vi "Halvorsen_ECD4_Fast.vi"(0 "tolerance":dbl=1e-13, 1 "Error Analysis":u16(ring)=4 items=["Max", "Max_Norm", "Norm", "Last Value", "Last Constant"], 3 "Шаг h, с":dbl=0.01, 4 "k":i32=4, 5 "Время, с":dbl=30.0, 7 "Hmax":dbl=1.0, 8 "b":dbl[](array[numeric])=[1.4, 1.4, 1.4], 10 "last_point_Thomas":dbl[](array[numeric])=[2.3727475682665875, 0.23609824454436878, 0.4447912442126299], 13 "Hmin":dbl=0.001, 15 "Points count":i32=2, 18 "n":i32[](array[numeric])=[2, 4, 6, 8, 10, 12, 14, 16, 18, 20, 22], 19 "Ext.Type":u16(ring) items=["FNode", "MathScript", "ECD8 Arrays", "ECD8 Fnode", "ECD8 FnodeDiv", "FNode Exp"]) -> (6 "Elapsed Time":dbl=0.006700851644382055, 12 "Number of steps":i32=211, 14 "Error Estimation":dbl=1.5745409996203077e-13, 17 "Rejected steps":i32=3)   [LabVIEW 2016]
uses:
  <vilib>/Analysis/_algsub.llb/Real Vector Norm.vi
  <vilib>/Analysis/5stat.llb/RMS (DBL).vi
  <vilib>/Analysis/NI_AALBase.lvlib
  <vilib>/Analysis/NI_AALPro.lvlib
panel:
  in  "Initial Conditions":dbl[](array[numeric])=[1.0, 0.0, 1.0]
  out "Last Value Reference":dbl[](array[numeric])=[2.3727475682668593, 0.2360982445442987, 0.44479124421215666] format="%#_15f"
  out "Rejected Steps":i32[](graph)=[0, 0, 0, 0, 0, 0, 0, 0, 0, 0, 0, 0, 0, 0, 0, 0, 0, 0, 0, 0, 0, 0, 0, 0, 0, 0, 0, 0, 0, 0, 0, 0, 0, 0, 0, 0, 0, 0, 0, 0, 0, 0, 0, 0, 0, 0, 0, 0, 0, 0, 0, 1, 0, 0, 0, 0, 0, 0, 0, 0, 0, 0, 0, 0, 0, 0, 0, 0, 0, 0, 0, 0, 0, 0, 0, 0, 0, 0, 0, 0, 0, 0, 0, 0, 0, 0, 1, 0, 0, 0, 0, 0, 0, 0, 0, 0, 0, 0, 0, 0, 0, 0, 0, 0, 0, 0, 0, 0, 0, 0, 0, 0, 0, 0, 0, 0, 0, 0, 0, 0, 0, 0, 0, 0, 0, 0, 0, 0, 0, 0, 0, 0, 0, 0, 0, 0, 0, 0, 0, 0, 0, 0, 0, 0, 0, 0, 0, 0, 0, 0, 0, 0, 0, 0, 0, 0, 0, 0, 0, 0, 0, 0, 0, 0, 0, 0, 0, 0, 0, 0, 0, 0, 0, 0, 0, 0, 0, 0, 0, 0, 0, 0, 0, 0, 0, 0, 0, 0, 1, 0, 0, 0, 0, 0, 0, 0, 0, 0, 0, 0, 0, 0, 0, 0, 0, 0, 0, 0, 0, 0, 0, 0]
  out "Last Value":dbl[](array[numeric])=[2.3727475682664667, 0.23609824454430522, 0.4447912442127084] format="%#_15f"
  out "Step time variation":dbl[](graph)=[0.006685207197733689, 0.006716496091030422]
  out "Real Error":dbl[][](graph)=[[0.0, 0.0, 0.0], [9.992007221626409e-16, 1.3877787807814457e-17, 4.6629367034256575e-15], [2.4424906541753444e-15, 3.122502256758253e-17, 6.661338147750939e-15], [-1.2212453270876722e-15, 2.914335439641036e-16, 5.551115123125783e-15], [-5.551115123125783e-15, -5.551115123125783e-17, 2.886579864025407e-15], [-5.10702591327572e-15, 2.7755575615628914e-16, 7.327471962526033e-15], [-7.771561172376096e-15, 1.1657341758564144e-15, 8.881784197001252e-15], [-6.661338147750939e-15, 2.886579864025407e-15, 9.103828801926284e-15], [-9.547918011776346e-15, -2.220446049250313e-16, 9.325873406851315e-15], [-8.215650382226158e-15, 2.886579864025407e-15, 1.1324274851176597e-14], [-7.771561172376096e-15, 2.6645352591003757e-15, 1.5987211554602254e-14], [-1.176836406102666e-14, 1.7763568394002505e-15, 7.327471962526033e-15], [-1.2878587085651816e-14, -1.5543122344752192e-15, 2.886579864025407e-15], [-1.1546319456101628e-14, 1.9984014443252818e-15, 9.769962616701378e-15], [-1.354472090042691e-14, -8.881784197001252e-16, 6.217248937900877e-15], [-2.1316282072803006e-14, -6.661338147750939e-15, 0.0], [-1.4654943925052066e-14, -4.218847493575595e-15, 8.881784197001252e-16], [-1.9539925233402755e-14, -6.661338147750939e-15, 4.884981308350689e-15], [-1.7763568394002505e-14, -1.1102230246251565e-14, 1.2434497875801753e-14], [-1.4654943925052066e-14, -1.3100631690576847e-14, 1.3766765505351941e-14], [-2.886579864025407e-14, -2.220446049250313e-14, 1.4210854715202004e-14], [-2.708944180085382e-14, -2.9976021664879227e-14, 2.1316282072803006e-14], [-3.1530333899354446e-14, -3.042011087472929e-14, 1.6431300764452317e-14], [-3.1530333899354446e-14, -3.219646771412954e-14, 1.8207657603852567e-14], [-3.5083047578154947e-14, -4.1522341120980855e-14, 2.353672812205332e-14], [-3.597122599785507e-14, -4.107825191113079e-14, 2.531308496145357e-14], [-3.6415315207705135e-14, -4.285460875053104e-14, 3.1530333899354446e-14], [-3.1530333899354446e-14, -4.529709940470639e-14, 3.241851231905457e-14], [-1.9539925233402755e-14, -4.285460875053104e-14, 2.708944180085382e-14], [-1.509903313490213e-14, -4.39648317751562e-14, 3.108624468950438e-14], [-2.398081733190338e-14, -4.973799150320701e-14, 2.708944180085382e-14], [-2.398081733190338e-14, -5.5067062021407764e-14, 3.597122599785507e-14], [-1.509903313490213e-14, -5.81756864903582e-14, 3.907985046680551e-14], [-2.7977620220553945e-14, -6.439293542825908e-14, 3.3306690738754696e-14], [-8.881784197001252e-15, -5.595524044110789e-14, 4.218847493575595e-14], [-9.769962616701378e-15, -5.3290705182007514e-14, 3.9968028886505635e-14], [-1.9539925233402755e-14, -5.950795411990839e-14, 3.574918139293004e-14], [-1.0658141036401503e-14, -6.261657858885883e-14, 3.68594044175552e-14], [-5.773159728050814e-15, -7.149836278586008e-14, 3.108624468950438e-14], [8.43769498715119e-15, -7.149836278586008e-14, 3.26405569239796e-14], [9.769962616701378e-15, -6.794564910705958e-14, 2.4202861936828413e-14], [1.7319479184152442e-14, -6.17284001691587e-14, 2.6645352591003757e-14], [2.1760371282653068e-14, -6.217248937900877e-14, 2.2648549702353193e-14], [2.531308496145357e-14, -5.551115123125783e-14, 2.731148640577885e-14], [2.6201263381153694e-14, -7.016609515630989e-14, 1.7985612998927536e-14], [4.218847493575595e-14, -7.283063041541027e-14, 1.2323475573339238e-14], [5.3734794391857577e-14, -7.327471962526033e-14, 6.328271240363392e-15], [6.394884621840902e-14, -6.972200594645983e-14, -2.1094237467877974e-15], [7.016609515630989e-14, -7.593925488436071e-14, -1.3766765505351941e-14], [8.304468224196171e-14, -6.616929226765933e-14, -2.2426505097428162e-14], [1.021405182655144e-13, -6.661338147750939e-14, -3.552713678800501e-14], [1.0791367799356522e-13, -6.616929226765933e-14, -5.1736392947532295e-14], [1.1501910535116622e-13, -5.1958437552457326e-14, -6.361577931102147e-14], [1.2256862191861728e-13, -3.952393967665557e-14, -7.51620987671231e-14], [1.318944953254686e-13, -3.907985046680551e-14, -8.304468224196171e-14], [1.3233858453531866e-13, -5.684341886080802e-14, -9.192646643896296e-14], [1.2789769243681803e-13, -7.904787935331115e-14, -9.880984919163893e-14], [1.361133428190442e-13, -7.815970093361102e-14, -1.0724754417879012e-13], [1.3566925360919413e-13, -8.08242361927114e-14, -1.1546319456101628e-13], [1.3811174426336947e-13, -8.260059303211165e-14, -1.1834977442504169e-13], [1.4477308241112041e-13, -7.638334409421077e-14, -1.0702549957386509e-13], [1.4588330543574557e-13, -6.661338147750939e-14, -1.0391687510491465e-13], [1.4432899320127035e-13, -4.796163466380676e-14, -9.947598300641403e-14], [1.3566925360919413e-13, -6.039613253960852e-14, -9.237055564881302e-14], [1.34781075189494e-13, -6.306066779870889e-14, -7.771561172376096e-14], [1.3433698597964394e-13, -4.1744385725905886e-14, -6.572520305780927e-14], [1.2756462552943049e-13, -5.3290705182007514e-14, -6.039613253960852e-14], [1.283417816466681e-13, -4.529709940470639e-14, -5.10702591327572e-14], [1.2784218128558678e-13, -4.1744385725905886e-14, -2.7533531010703882e-14], [1.2423395645555502e-13, -4.3520742565306136e-14, -1.865174681370263e-14], [1.2059797604990763e-13, -5.240252676230739e-14, -1.2434497875801753e-14], [1.168370955539899e-13, -5.240252676230739e-14, 7.549516567451064e-15], [1.1368683772161603e-13, -4.973799150320701e-14, 2.6645352591003757e-14], [1.1013412404281553e-13, -2.930988785010413e-14, 4.618527782440651e-14], [1.0680345496894006e-13, -6.217248937900877e-14, 5.573319583618286e-14], [1.0169642905566434e-13, -7.37188088351104e-14, 7.038813976123492e-14], [9.348077867343818e-14, -6.661338147750939e-14, 8.126832540256146e-14], [8.926193117986259e-14, -7.105427357601002e-14, 8.72635297355373e-14], [8.004708007547379e-14, -5.1514348342607263e-14, 9.814371537686384e-14], [7.527312106958561e-14, -6.661338147750939e-14, 9.792167077193881e-14], [6.750155989720952e-14, -3.197442310920451e-14, 1.0458300891968975e-13], [6.283862319378386e-14, -4.796163466380676e-14, 1.028066520802895e-13], [5.417888360170764e-14, -2.4868995751603507e-14, 1.0624834345662748e-13], [4.9960036108132044e-14, -1.7763568394002505e-15, 1.0802470029602773e-13], [5.484501741648273e-14, 8.881784197001252e-15, 1.0758061108617767e-13], [5.5067062021407764e-14, 2.842170943040401e-14, 1.0608181000293371e-13], [6.217248937900877e-14, 1.5987211554602254e-14, 1.0330625244137082e-13], [6.750155989720952e-14, 3.8191672047105385e-14, 1.010788674982166e-13], [7.194245199571014e-14, 3.9968028886505635e-14, 9.781064846947629e-14], [6.52811138479592e-14, 6.838973831690964e-14, 9.320322291728189e-14], [6.039613253960852e-14, 9.769962616701378e-14, 8.709699628184353e-14], [7.016609515630989e-14, 1.199040866595169e-13, 8.115730310009894e-14], [7.815970093361102e-14, 1.1191048088221578e-13, 7.494005416219807e-14], [8.482103908136196e-14, 1.0302869668521453e-13, 6.661338147750939e-14], [9.414691248821327e-14, 8.43769498715119e-14, 6.139533326177116e-14], [1.0347278589506459e-13, 7.904787935331115e-14, 5.4289905904170155e-14], [9.947598300641403e-14, 7.283063041541027e-14, 4.5630166312093934e-14], [8.482103908136196e-14, 9.769962616701378e-14, 3.26405569239796e-14], [8.748557434046234e-14, 1.0302869668521453e-13, 2.4202861936828413e-14], [7.505107646466058e-14, 9.325873406851315e-14, 1.4876988529977098e-14], [7.815970093361102e-14, 8.393286066166183e-14, 4.6629367034256575e-15], [7.327471962526033e-14, 8.304468224196171e-14, -2.886579864025407e-15], [6.616929226765933e-14, 7.815970093361102e-14, -8.215650382226158e-15], [6.394884621840902e-14, 6.394884621840902e-14, -1.3100631690576847e-14], [5.773159728050814e-14, 5.595524044110789e-14, -2.1538326677728037e-14], [3.907985046680551e-14, 5.3290705182007514e-14, -2.2426505097428162e-14], [3.552713678800501e-14, 4.529709940470639e-14, -2.19824158875781e-14], [3.419486915845482e-14, 2.6645352591003757e-14, -2.0650148258027912e-14], [3.863576125695545e-14, 2.531308496145357e-14, -2.375877272697835e-14], [2.1760371282653068e-14, 3.4638958368304884e-14, -3.2862601528904634e-14], [1.687538997430238e-14, 2.353672812205332e-14, -2.2870594307278225e-14], [3.9968028886505635e-15, 3.064215547965432e-14, -2.708944180085382e-14], [6.661338147750939e-16, 3.1308289294429414e-14, -2.5091040356528538e-14], [1.3322676295501878e-15, 2.708944180085382e-14, -1.7541523789077473e-14], [-3.9968028886505635e-15, 2.7977620220553945e-14, -2.2426505097428162e-14], [-4.440892098500626e-16, 2.7755575615628914e-14, -2.020605904817785e-14], [-2.6645352591003757e-15, 3.086420008457935e-14, -3.1530333899354446e-14], [3.552713678800501e-15, 2.6201263381153694e-14, -2.4424906541753444e-14], [5.329070518200751e-15, 2.7755575615628914e-14, -1.9984014443252818e-14], [8.659739592076221e-15, 2.6756374893466273e-14, -1.687538997430238e-14], [8.43769498715119e-15, 3.175237850427948e-14, -3.2862601528904634e-14], [9.547918011776346e-15, 3.4638958368304884e-14, -3.108624468950438e-14], [1.7985612998927536e-14, 3.26405569239796e-14, -2.7533531010703882e-14], [2.1871393585115584e-14, 3.2862601528904634e-14, -1.865174681370263e-14], [2.7478019859472624e-14, 3.275157922644212e-14, -9.325873406851315e-15], [3.325117958752344e-14, 3.0309088572266774e-14, 4.440892098500626e-15], [3.6137759451548845e-14, 2.7533531010703882e-14, 1.1102230246251565e-14], [3.902433931557425e-14, 2.525757381022231e-14, 1.6431300764452317e-14], [4.1799896877137144e-14, 2.2065682614424986e-14, 2.1760371282653068e-14], [4.3770542745846797e-14, 1.940114735532461e-14, 1.7319479184152442e-14], [4.601874437071274e-14, 1.6014967130217883e-14, 2.6201263381153694e-14], [4.718447854656915e-14, 1.2692971673722298e-14, 2.4424906541753444e-14], [4.835021272242557e-14, 7.827072323607354e-15, 3.774758283725532e-14], [4.85722573273506e-14, 9.43689570931383e-16, 4.6629367034256575e-14], [4.7600812180803587e-14, -5.773159728050814e-15, 5.3290705182007514e-14], [4.696243394164412e-14, -1.3877787807814457e-14, 7.327471962526033e-14], [4.4353409833775004e-14, -2.4369395390522186e-14, 8.215650382226158e-14], [3.835820550079916e-14, -3.652633751016765e-14, 8.659739592076221e-14], [3.36952687973735e-14, -4.7406523151494184e-14, 8.570921750106208e-14], [2.531308496145357e-14, -5.81756864903582e-14, 8.615330671091215e-14], [1.8540724511240114e-14, -6.872280522429719e-14, 9.192646643896296e-14], [1.1324274851176597e-14, -7.815970093361102e-14, 9.50350909079134e-14], [4.773959005888173e-15, -9.092726571680032e-14, 1.0391687510491465e-13], [-2.1094237467877974e-15, -1.0402789740737717e-13, 1.1723955140041653e-13], [-1.5765166949677223e-14, -1.2312373343092986e-13, 1.1857181902996672e-13], [-3.2862601528904634e-14, -1.4199752484955752e-13, 1.2079226507921703e-13], [-4.463096558993129e-14, -1.5831780331154732e-13, 1.2789769243681803e-13], [-6.283862319378386e-14, -1.7563728249569976e-13, 1.3322676295501878e-13], [-8.038014698286133e-14, -1.9340085088970227e-13, 1.2434497875801753e-13], [-1.0591527654923993e-13, -2.0794477251229182e-13, 1.0702549957386509e-13], [-1.383337888682945e-13, -2.199351811782435e-13, 8.570921750106208e-14], [-1.6653345369377348e-13, -2.2687407508215074e-13, 8.704148513061227e-14], [-1.949551631241775e-13, -2.3397950243975174e-13, 8.970602038971265e-14], [-2.2648549702353193e-13, -2.410571742217371e-13, 9.992007221626409e-14], [-2.6334490144108713e-13, -2.4702462297909733e-13, 8.171241461241152e-14], [-2.9265478929119126e-13, -2.50716114535976e-13, 8.970602038971265e-14], [-3.277378368693462e-13, -2.545741395465484e-13, 1.0036416142611415e-13], [-3.597122599785507e-13, -2.581268532253489e-13, 1.163513729807164e-13], [-3.8413716652030416e-13, -2.602362769721367e-13, 1.1546319456101628e-13], [-4.078959392472825e-13, -2.62234678416462e-13, 1.199040866595169e-13], [-4.289901767151605e-13, -2.62234678416462e-13, 9.059419880941277e-14], [-4.511946372076636e-13, -2.575717417130363e-13, 5.5067062021407764e-14], [-4.662936703425657e-13, -2.552402733613235e-13, 7.105427357601002e-15], [-4.745093207247919e-13, -2.5268676040468563e-13, -4.085620730620576e-14], [-4.815037257799304e-13, -2.489120021209601e-13, -8.08242361927114e-14], [-4.833911049217932e-13, -2.502442697505103e-13, -1.1457501614131615e-13], [-4.843903056439558e-13, -2.475797344914099e-13, -1.4832579608992091e-13], [-4.796163466380676e-13, -2.5224267119483557e-13, -1.865174681370263e-13], [-4.726219415829291e-13, -2.4846791291111003e-13, -2.5845992013273644e-13], [-4.62907490117459e-13, -2.475797344914099e-13, -3.090860900556436e-13], [-4.5086157030027607e-13, -2.4003021792395884e-13, -3.9523939676655573e-13], [-4.3623438195083963e-13, -2.313704783318826e-13, -4.4231285301066237e-13], [-4.1983083676200295e-13, -2.2515322939398175e-13, -4.627409566637652e-13], [-3.990696662015125e-13, -2.0028423364237824e-13, -5.160316618457728e-13], [-3.79585252119341e-13, -1.6786572132332367e-13, -5.586642259913788e-13], [-3.6270986214503864e-13, -1.341149413747189e-13, -6.048495038157853e-13], [-3.446132268436486e-13, -8.570921750106208e-14, -6.421529974431905e-13], [-3.326228181776969e-13, -1.865174681370263e-14, -6.679101716144942e-13], [-3.3284486278262193e-13, 6.616929226765933e-14, -6.918909889463976e-13], [-3.398392678377604e-13, 1.7053025658242404e-13, -7.291944825738028e-13], [-3.6348701826227625e-13, 2.8466118351389014e-13, -7.633893517322576e-13], [-4.050093593832571e-13, 4.0234482412415673e-13, -7.709388682997087e-13], [-4.531930386519889e-13, 5.258016244624741e-13, -7.931433287922118e-13], [-5.131450819817474e-13, 6.346034808757395e-13, -8.109068971862143e-13], [-5.799805080641818e-13, 7.371880883511039e-13, -8.326672684688674e-13], [-6.459277557269161e-13, 8.175682353339653e-13, -8.402167850363185e-13], [-7.001066393286237e-13, 8.921752225887758e-13, -8.624212455288216e-13], [-7.502887200416808e-13, 9.374723219934822e-13, -8.557599073810707e-13], [-7.913669719528116e-13, 9.832135106080386e-13, -8.419931418757187e-13], [-8.022471575941381e-13, 1.007194327939942e-12, -8.231193504570911e-13], [-8.033573806187633e-13, 1.0158540675320182e-12, -7.902567489281864e-13], [-7.902567489281864e-13, 1.0114131754335176e-12, -7.538414337204813e-13], [-7.620570841027074e-13, 9.9253938401489e-13, -7.049916206369744e-13], [-7.225331444260519e-13, 9.65227897609111e-13, -6.481482017761664e-13], [-6.497025140106416e-13, 9.319212068703564e-13, -5.915268275202834e-13], [-5.644373857194296e-13, 8.967271369897389e-13, -5.426770144367765e-13], [-4.902744876744691e-13, 8.524292383071952e-13, -4.947153797729698e-13], [-4.1966430330830917e-13, 8.066880496926387e-13, -4.455324997820753e-13], [-3.299582829185965e-13, 7.603917495657697e-13, -4.034550471487819e-13], [-2.4158453015843406e-13, 7.093770015842438e-13, -3.672617765460018e-13], [-1.580957587066223e-13, 6.575850974854802e-13, -3.377298440909726e-13], [-5.062616992290714e-14, 6.074585279236544e-13, -3.207434318142077e-13], [4.263256414560601e-14, 5.561107130347409e-13, -3.161360062620133e-13], [1.283417816466681e-13, 5.040690087554367e-13, -3.2229774404868294e-13], [2.0472512574087887e-13, 4.4883541328033516e-13, -3.3889557826682903e-13], [2.6556534749033744e-13, 3.8989644846054716e-13, -3.6187719487656977e-13], [3.157474282033945e-13, 3.2633618030075695e-13, -3.9163117193652397e-13], [3.4638958368304884e-13, 2.5711377471537844e-13, -4.2539582967293654e-13], [3.859135233597044e-13, 1.8274270985330077e-13, -4.619638005465276e-13], [3.956834859764058e-13, 1.0211276268989877e-13, -5.017652959793395e-13], [3.943512183468556e-13, 1.712519015484304e-14, -5.417333248658451e-13], [3.9257486150745535e-13, -6.522560269672795e-15, -5.517253320874715e-13]]
  out "Step Variation":dbl[](graph)=[0.01, 0.023360677996708375, 0.05456832298719971, 0.10609865677759227, 0.14228685817737252, 0.1433521858258461, 0.13912016368248273, 0.1353848978239948, 0.1348787008039935, 0.13789794946241468, 0.14183965168589427, 0.1389018246685753, 0.13480655511664044, 0.1352937955188443, 0.14083631069515853, 0.15054302015732818, 0.15354936807919295, 0.15012909437801925, 0.15233158646615488, 0.16195221907261806, 0.1859888941921947, 0.19081476436473468, 0.16882309271455131, 0.16110756221534117, 0.15751551557922944, 0.15515566263423652, 0.1537986192378969, 0.15441647648808968, 0.15703348889728966, 0.16223661244468615, 0.16523261129770903, 0.1575552847464681, 0.14923788348804234, 0.14420094794209656, 0.14333043693757236, 0.14305599030596625, 0.1451932462186197, 0.1484158449420317, 0.15105915525521163, 0.15267209809470114, 0.15128993514268424, 0.1473508980423149, 0.14417110851040923, 0.14259673520710134, 0.1438612133690481, 0.14531637887383417, 0.1489824606828707, 0.15335475631763087, 0.1583176965097996, 0.1645478155214016, 0.1758092639086622, 0.1662066741033067, 0.1471159764326851, 0.1367282453140493, 0.13035995246764745, 0.12717631788307218, 0.12761153374775996, 0.13218596626534898, 0.1395535058928262, 0.1359873295729682, 0.1279072153561344, 0.12677916749215723, 0.13020671862805994, 0.14054161466738815, 0.14955735646322033, 0.1422870923630447, 0.13947030152822443, 0.1425137619209431, 0.14861606101153554, 0.15532871545503943, 0.16063336757924904, 0.16156986300229476, 0.15420612102053258, 0.1452179402961989, 0.13922466410526793, 0.13618167321476882, 0.13478266135199252, 0.13483812596599676, 0.1368349300001295, 0.1419973850154061, 0.1492979861408155, 0.1630793688516221, 0.1698407314481118, 0.1660731905847401, 0.16476318145002147, 0.17023890658894714, 0.17794557645431167, 0.15417389965318076, 0.14164279375448932, 0.13699467420144448, 0.14016009907464672, 0.14454490990645175, 0.13059324979206005, 0.12253189529550425, 0.1201054691030008, 0.12208443771041655, 0.1268938879187612, 0.13135378363117228, 0.13149948182226284, 0.13091376094679263, 0.1330358218423598, 0.13498918498691118, 0.134693349945233, 0.1332797222087208, 0.1327545271092479, 0.132096286825721, 0.12572137094659197, 0.11851952468371733, 0.11440885990029541, 0.11408975301000251, 0.11845938663500437, 0.1251657972697687, 0.11744274061194553, 0.11116682029079179, 0.11109183499278635, 0.11563403836804881, 0.12843660419635064, 0.1340781134326106, 0.12308149559662285, 0.121269099319311, 0.12397097627136096, 0.1310044455798987, 0.14256647877408143, 0.15612558917515526, 0.1559767909870482, 0.1516395775231047, 0.15061109839379794, 0.15131873674559188, 0.15303037557568117, 0.15537721190750214, 0.15765681556191427, 0.16079007115021313, 0.16385724409617003, 0.167421072233169, 0.1705799765382728, 0.17136763902468344, 0.16834897464401802, 0.16344776456145238, 0.15906244550119522, 0.15566817976109593, 0.15384896253401684, 0.15397043019905826, 0.15647351646131896, 0.162778286355558, 0.17312680493100446, 0.17301716184922508, 0.16211595058856945, 0.156911165553237, 0.1572960348891089, 0.1621783969662183, 0.16988978762207912, 0.1676270098812039, 0.15942001429121724, 0.15559916575909497, 0.15555986759313123, 0.1559835273600667, 0.1507770825869849, 0.14519292747781615, 0.1433104622596264, 0.14815336806507956, 0.1568099336449324, 0.14420289290775362, 0.1355769624824643, 0.1343908665158623, 0.1370423708466838, 0.13629799178478536, 0.12965040110128848, 0.12412220297706678, 0.12165762374815889, 0.12108927036893419, 0.12229191822314137, 0.1249944269950167, 0.12751852881829193, 0.12884740536200978, 0.13001514453120236, 0.13295980367479468, 0.13840032844181696, 0.14741206326398376, 0.1600655659399263, 0.16646454630924873, 0.15939804241832492, 0.1539502667088633, 0.15155926283142948, 0.14757446042942224, 0.13541405056970915, 0.1283102292451462, 0.12813003375040924, 0.14225861622847752, 0.1379919455900096, 0.11953673896290772, 0.1151409444583287, 0.11697515743692918, 0.12465131478568296, 0.13338397902464036, 0.1250281665230314, 0.12183451816436883, 0.12393101719177703, 0.12916307570698296, 0.13739294100052019, 0.14654556714718814, 0.15040081725418902, 0.15046036573986937, 0.15011424337824786, 0.15087157526841347, 0.1526751737514233, 0.1550753687685979, 0.15872031300368974, 0.16265538427893264, 0.16696159138984856, 0.17040820371236481, 0.04907266583554204, 0.0]
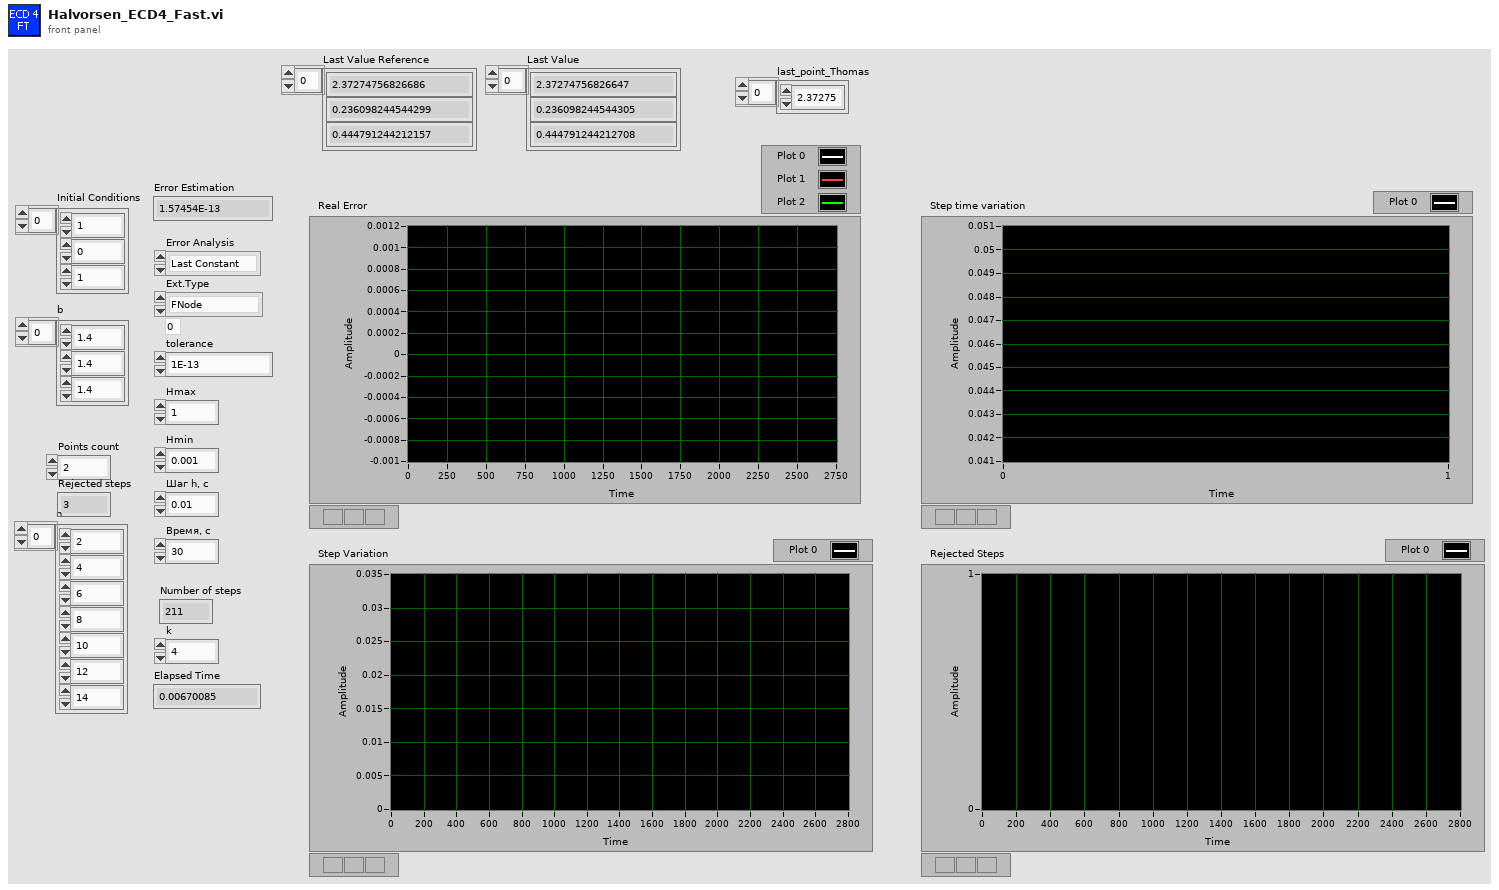
[diagram p1: front panel]
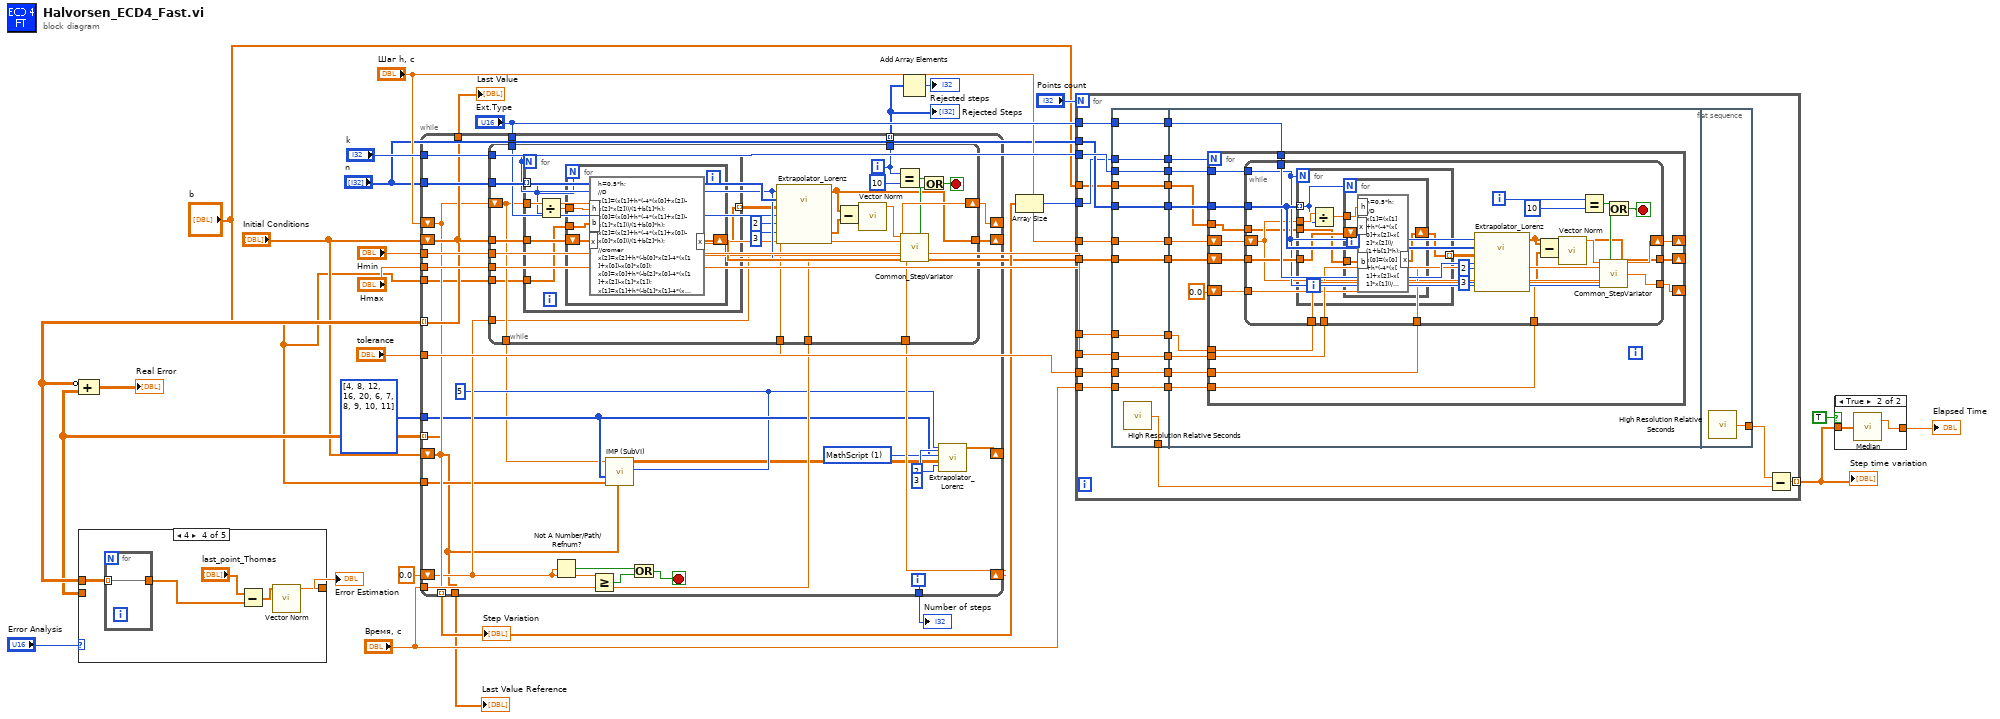
[diagram p0: block diagram]
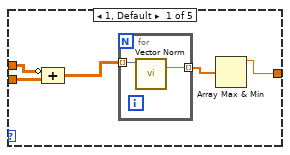
[diagram p2: hidden frame]
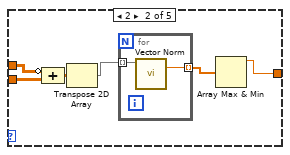
[diagram p3: hidden frame]
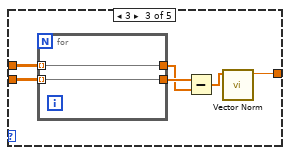
[diagram p4: hidden frame]
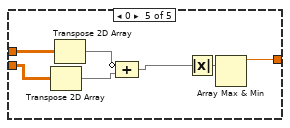
[diagram p5: hidden frame]
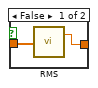
[diagram p6: hidden frame]
diagram:
  n1 = while {
    shift-right: [w50] -> _
    shift-left: "Initial Conditions" -> [w43]
    tunnel: "n" -> [w57]
    tunnel: "k" -> [w55]
    tunnel: "Ext.Type" -> [w46]
    shift-right: [w54] -> _
    shift-left: "Шаг h, с" -> [w37]
    shift-right: [w45] -> _
    shift-left: 0.0 -> [w36]
    tunnel: [w37] -> w13 mode=indexing
    tunnel: "Время, с" -> [w44]
    tunnel: [w56] -> w23
    tunnel: "tolerance" -> [w51]
    tunnel: "Hmin" -> [w53]
    tunnel: "Hmax" -> [w52]
    tunnel: [w43] -> w6 mode=indexing
    shift-right: [w49] -> _
    shift-left: "Initial Conditions" -> [w30]
    tunnel: i32[] [4, 8, 12, 16, 20, 6, 7, 8, 9, 10, 11] ("n 2") -> [w34]
    tunnel: [w30] -> w5 mode=indexing
    tunnel: [w43] -> w11
    tunnel: [w42] -> w10 mode=indexing
    tunnel: [w30] -> w4
    tunnel: "b" -> [w31]
    tunnel: "b" -> [w35]
    i -> [w56]
    stop <- w38 stop-if-true
    w41 = u16 1 items=["FNode", "MathScript", "ECD8 Arrays", "ECD8 Fnode", "ECD8 FnodeDiv"] ("Ext.Type")
    w33 = 5
    n2 = while {
      tunnel: w57 -> [w82]
      tunnel: w55 -> [w81]
      tunnel: w53 -> [w79]
      tunnel: w52 -> [w78]
      tunnel: w51 -> [w77]
      tunnel: [w60] -> w50
      tunnel: w46 -> [w73]
      tunnel: [w64] -> w45
      tunnel: w44 -> [w72]
      tunnel: w43 -> [w71]
      shift-right: [w80] -> w54
      shift-left: w37 -> [w66]
      tunnel: [w66] -> w32
      tunnel: [w65] -> w42
      tunnel: w36 -> [w63]
      tunnel: w35 -> [w62]
      i -> [w65]
      stop <- w68 stop-if-true
      n3 = for {
        N: w81 -> [_]
        tunnel: w82 -> [w85] mode=indexing
        tunnel: w66 -> [w86]
        tunnel: w71 -> [w88]
        tunnel: [w87] -> w74 mode=indexing
        tunnel: w62 -> [w83]
        n4 = Divide(x=w86, y=w85) -> (x/y=w84:dbl)
        n5 = for {
          N: w85 -> [_]
          shift-right: [w91] -> w87
          shift-left: w88 -> [w92]
          tunnel: w84 -> [w90]
          tunnel: w83 -> [w89]
          n6 = formula code="h=0.5*h;\n//D\nx[1]=(x[1]+h*(-4*(x[0]+x[2])-x[2]*x[2]))/(1+b[1]*h);\nx[0]=(x[0]+h*(-4*(x[1]+x[2])-x[1]*x[1]))/(1+b[0]*h);\nx[2]=(x[2]+h*(-4*(x[1]+x[0])-x[0]*x[0]))/(1+b[2]*h);\n//cromer\nx[2]=x[2]+h*(-b[0]*x[2]-4*(x[1]+x[0])-x[0]*x[0]);\nx[0]=x[0]+h*(-b[2]*x[0]-4*(x[1]+x[2])-x[1]*x[1]);\nx[1]=x[1]+h*(-b[1]*x[1]-4*(x[0]+x[2])-x[2]*x[2]);"("x"=w92, "h"=w90, "b"=w89) -> ("x"=w91:dbl[])
        }
      }
      n7 = call "Extrapolator_Lorenz.vi"("Порядок экстраполятора"=2 ("input variable"), "Dimension"=3 ("input variable"), "Ext.Type"=w73, "Х - нач. условия"=w74, "n"=w82, "k"=w81) -> ("TPrev"=w59:dbl[], "Tout"=w60:dbl[])  [unwired: 4 in]
      n8 = Subtract(x=w60, y=w59) -> (x-y=w61:dbl[])
      n9 = call-poly <vilib>:"Vector Norm.vi"("Input Vector"=w61) -> ("norm"=w58:dbl)  [unwired: 9 in, 1 out]
      n10 = Equal?(x=w65, y=10) -> (x = y?=w70:bool)
      n11 = call "Common_StepVariator.vi"("err"=w58, "tolerance"=w77, "Hmax"=w78, "Шаг h, с"=w66, "Current time"=w63, "k"=w81, "Hmin"=w79, "tmax"=w72) -> ("Hnew"=w80:dbl, "New time"=w64:dbl, "stop"=w67:bool)  [unwired: 4 in, 1 out]
      n12 = Or(x=w70, y=w67) -> (x .or. y?=w68:bool)
    }
    n13 = Not A Number/Path/Refnum?(number/path/refnum=w36) -> (NaN/Path/Refnum?=w40:bool)
    n14 = Greater Or Equal?(x=w36, y=w44) -> (x >= y?=w39:bool)
    n15 = call "IMP (SubVI).vi"("Initial Conditions in"=w30, "b"=w31, "n in"=w34, "Numeric"=w33, "Шаг h, с"=w32) -> ("Initial Conditions out"=w29:dbl[][])  [unwired: 6 in]
    n16 = Or(x=w40, y=w39) -> (x .or. y?=w38:bool)
    n17 = call "Extrapolator_Lorenz.vi"("Порядок экстраполятора"=2, "Dimension"=3, "Ext.Type"=w41, "Х - нач. условия"=w29, "n"=w34, "k"=w33) -> ("Tout"=w49:dbl[])  [unwired: 4 in, 1 out]
  }
  "Step Variation" <- w13
  "Number of steps" <- w23
  "Last Value" <- w11
  "Rejected Steps" <- w10
  "Last Value Reference" <- w4
  n18 = Compound Arithmetic op=ADD(invert w6, w5) -> (→"Real Error":dbl[][])
  n19 = case shown="4" "Error Analysis" {
    tunnel: w5 -> [w94 w102 w111 _ w122]
    tunnel: [w96 w104 w113 w120 w127] -> w8
    tunnel: w6 -> [w95 w103 w112 w119 w123]
    frame 1, Default {
      n20 = Compound Arithmetic op=ADD(invert w95, w94) -> (w93:dbl[][])
      n21 = for {
        tunnel: [w99] -> w97 mode=indexing
        tunnel: w93 -> [w98] mode=indexing
        n22 = call-poly <vilib>:"Vector Norm.vi"("Input Vector"=w98) -> ("norm"=w99:dbl)  [unwired: 9 in, 1 out]
      }
      n23 = Array Max & Min(array=w97) -> (max value=w96:dbl)  [unwired: 3 out]
    }
    frame 2 {
      n24 = Compound Arithmetic op=ADD(invert w103, w102) -> (w101:dbl[][])
      n25 = Transpose 2D Array(2D array=w101) -> (transposed array=w100:dbl[][])
      n26 = for {
        tunnel: [w107] -> w105 mode=indexing
        tunnel: w100 -> [w106] mode=indexing
        n27 = call-poly <vilib>:"Vector Norm.vi"("Input Vector"=w106) -> ("norm"=w107:dbl)  [unwired: 9 in, 1 out]
      }
      n28 = Array Max & Min(array=w105) -> (max value=w104:dbl)  [unwired: 3 out]
    }
    frame 3 {
      n29 = for {
        tunnel: w112 -> [w115] mode=indexing
        tunnel: [w115] -> w109
        tunnel: w111 -> [w114] mode=indexing
        tunnel: [w114] -> w110
      }
      n30 = Subtract(x=w110, y=w109) -> (x-y=w108:dbl[])
      n31 = call-poly <vilib>:"Vector Norm.vi"("Input Vector"=w108) -> ("norm"=w113:dbl)  [unwired: 9 in, 1 out]
    }
    frame 4 {
      n32 = for {
        tunnel: w119 -> [w121] mode=indexing
        tunnel: [w121] -> w118
      }
      n33 = Subtract(x="last_point_Thomas", y=w118) -> (x-y=w117:dbl[])
      n34 = call-poly <vilib>:"Vector Norm.vi"("Input Vector"=w117) -> ("norm"=w120:dbl)  [unwired: 9 in, 1 out]
    }
    frame 0 {
      n35 = Transpose 2D Array(2D array=w122) -> (transposed array=w125:dbl[][])
      n36 = Transpose 2D Array(2D array=w123) -> (transposed array=w126:dbl[][])
      n37 = Compound Arithmetic op=ADD(invert w126, w125) -> (w124:dbl[][])
      n38 = Absolute Value(x=w124) -> (abs(x)=w128:dbl[][])
      n39 = Array Max & Min(array=w128) -> (max value=w127:dbl)  [unwired: 3 out]
    }
  }
  "Error Estimation" <- w8
  n40 = Add Array Elements(numeric array=w10) -> (sum=→"Rejected steps":i32)
  n41 = Array Size(array=w13) -> (size(s)=w22:i32)
  n42 = for {
    N: "Points count" -> [_]
    tunnel: "k" -> [w153]
    tunnel: "n" -> [w152]
    tunnel: "Ext.Type" -> [w132]
    tunnel: "Initial Conditions" -> [w151]
    tunnel: w22 -> [w150]
    tunnel: [w143] -> w20 mode=indexing
    tunnel: "Шаг h, с" -> [w134]
    tunnel: "Hmin" -> [w142]
    tunnel: "Hmax" -> [w139]
    tunnel: "tolerance" -> [w138]
    tunnel: "Время, с" -> [w136]
    tunnel: "b" -> [w129]
    n43 = flat-sequence {
      tunnel: w150 -> [w162]
      tunnel: w151 -> [w163]
      tunnel: w152 -> [w164]
      tunnel: w153 -> [w165]
      tunnel: [w165] -> w149
      tunnel: [w164] -> w148
      tunnel: [w163] -> w147
      tunnel: [w162] -> w146
      tunnel: [w161] -> w144
      tunnel: w142 -> [w160]
      tunnel: [w160] -> w141
      tunnel: w139 -> [w159]
      tunnel: [w159] -> w140
      tunnel: w138 -> [w158]
      tunnel: [w158] -> w137
      tunnel: w136 -> [w157]
      tunnel: [w157] -> w135
      tunnel: w134 -> [w156]
      tunnel: [w156] -> w133
      tunnel: w132 -> [w155]
      tunnel: [w155] -> w131
      tunnel: [w154] -> w130
      tunnel: w129 -> [w154]
      tunnel: w149 -> [w177]
      tunnel: w148 -> [w176]
      tunnel: w147 -> [w175]
      tunnel: w146 -> [w174]
      tunnel: w141 -> [w172]
      tunnel: w140 -> [w171]
      tunnel: w137 -> [w170]
      tunnel: w135 -> [w169]
      tunnel: w133 -> [w168]
      tunnel: w131 -> [w167]
      tunnel: w130 -> [w166]
      tunnel: [w227] -> w145
      frame #0 {
        n44 = call <vilib>:"High Resolution Relative Seconds.vi"() -> ("relative seconds"=w161:dbl)
      }
      frame #1 {
        n45 = for {
          N: w174 -> [_]
          shift-right: [w188] -> _
          shift-left: w175 -> [w179]
          tunnel: w176 -> [w191]
          tunnel: w177 -> [w187]
          tunnel: w167 -> [w190]
          shift-right: [w189] -> _
          shift-left: w168 -> [w182]
          tunnel: w172 -> [w186]
          tunnel: w171 -> [w185]
          tunnel: w170 -> [w184]
          shift-right: [w181] -> _
          shift-left: 0.0 -> [w180]
          tunnel: w169 -> [w183]
          tunnel: w166 -> [w178]
          n46 = while {
            tunnel: w191 -> [w216]
            tunnel: w190 -> [w215]
            tunnel: w179 -> [w214]
            tunnel: [w193] -> w188
            tunnel: w187 -> [w209]
            tunnel: w186 -> [w208]
            tunnel: w185 -> [w207]
            tunnel: w184 -> [w206]
            tunnel: w180 -> [w205]
            tunnel: w183 -> [w204]
            shift-right: [w210] -> w189
            shift-left: w182 -> [w197]
            tunnel: [w198] -> w181
            tunnel: w178 -> [w196]
            i -> [w200]
            stop <- w201 stop-if-true
            n47 = for {
              N: w209 -> [_]
              tunnel: w216 -> [w219] mode=indexing
              tunnel: w197 -> [w220]
              tunnel: w214 -> [w222]
              tunnel: [w221] -> w211 mode=indexing
              tunnel: w196 -> [w217]
              n48 = Divide(x=w220, y=w219) -> (x/y=w218:dbl)
              n49 = for {
                N: w219 -> [_]
                shift-right: [w225] -> w221
                shift-left: w222 -> [w226]
                tunnel: w218 -> [w224]
                tunnel: w217 -> [w223]
                n50 = formula code="h=0.5*h;\n//D\nx[1]=(x[1]+h*(-4*(x[0]+x[2])-x[2]*x[2]))/(1+b[1]*h);\nx[0]=(x[0]+h*(-4*(x[1]+x[2])-x[1]*x[1]))/(1+b[0]*h);\nx[2]=(x[2]+h*(-4*(x[1]+x[0])-x[0]*x[0]))/(1+b[2]*h);\n//cromer\nx[2]=x[2]+h*(-b[0]*x[2]-4*(x[1]+x[0])-x[0]*x[0]);\nx[0]=x[0]+h*(-b[2]*x[0]-4*(x[1]+x[2])-x[1]*x[1]);\nx[1]=x[1]+h*(-b[1]*x[1]-4*(x[0]+x[2])-x[2]*x[2]);"("x"=w226, "h"=w224, "b"=w223) -> ("x"=w225:dbl[])
              }
            }
            n51 = call "Extrapolator_Lorenz.vi"("Порядок экстраполятора"=2 ("input variable"), "Dimension"=3 ("input variable"), "Ext.Type"=w215, "Х - нач. условия"=w211, "n"=w216, "k"=w209) -> ("TPrev"=w192:dbl[], "Tout"=w193:dbl[])  [unwired: 4 in]
            n52 = Subtract(x=w193, y=w192) -> (x-y=w195:dbl[])
            n53 = call-poly <vilib>:"Vector Norm.vi"("Input Vector"=w195) -> ("norm"=w194:dbl)  [unwired: 9 in, 1 out]
            n54 = Equal?(x=w200, y=10) -> (x = y?=w202:bool)
            n55 = call "Common_StepVariator.vi"("err"=w194, "tolerance"=w206, "Hmax"=w207, "Шаг h, с"=w197, "Current time"=w205, "k"=w209, "Hmin"=w208, "tmax"=w204) -> ("Hnew"=w210:dbl, "New time"=w198:dbl, "stop"=w199:bool)  [unwired: 4 in, 1 out]
            n56 = Or(x=w202, y=w199) -> (x .or. y?=w201:bool)
          }
        }
      }
      frame #2 {
        n57 = call <vilib>:"High Resolution Relative Seconds.vi"() -> ("relative seconds"=w227:dbl)
      }
    }
    n58 = Subtract(x=w145, y=w144) -> (x-y=w143:dbl)
  }
  "Step time variation" <- w20
  n59 = case shown="True" TRUE {
    tunnel: w20 -> [w228 w231]
    tunnel: [w229 w230] -> w19
    frame False {
      n60 = call-poly <vilib>:"RMS.vi"("X"=w228) -> ("rms value"=w229:dbl)  [unwired: 1 out]
    }
    frame True {
      n61 = call <vilib>:"Median.vi"("X"=w231) -> ("median"=w230:dbl)  [unwired: 1 out]
    }
  }
  "Elapsed Time" <- w19
